vi "Profile_minus_Mean.vi"() -> (0 "New Values In":string[][](array[string])=[["Test data5"]], 1 "New Chs In":string[](array[string])=["30-10-03:New:Channel new5"])   [LabVIEW 2011]
uses:
  Results_plotter_Global.vi
  <vilib>/Analysis/NI_AALBase.lvlib
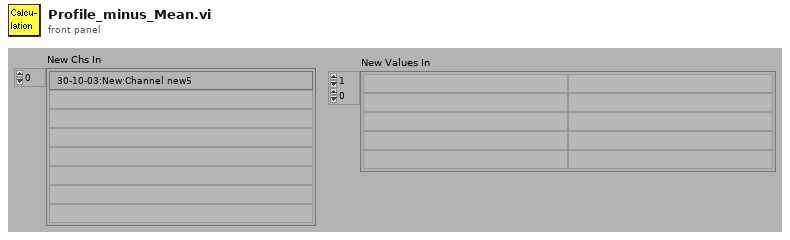
[diagram p1: front panel]
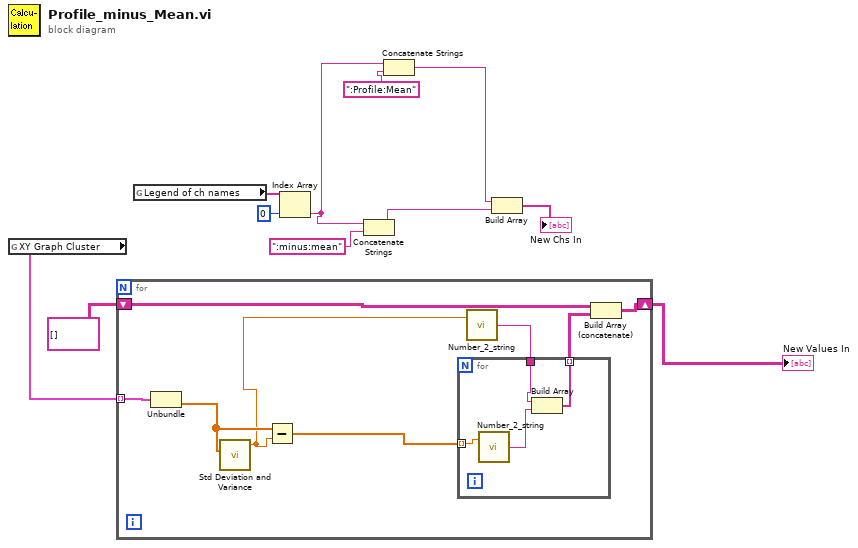
[diagram p0: block diagram]
diagram:
  n1 = global read "Results_plotter_Global.vi" "XY Graph Cluster"() -> (w9:cluster{dbl[], dbl[]}[])
  n2 = for {
    tunnel: w9 -> [w19] mode=indexing
    shift-right: [w15] -> w4
    shift-left: string[][] [] -> [w17]
    n3 = Unbundle(w19) -> (w18:dbl[])  [unwired: 1 out]
    n4 = call <vilib>:"Std Deviation and Variance.vi"("X"=w18) -> ("mean"=w14:dbl)  [unwired: 1 in, 2 out]
    n5 = Subtract(x=w18, y=w14) -> (x-y=w12:dbl[])
    n6 = call "Number_2_string.vi"("number"=w14) -> ("String"=w13:string)  [unwired: 1 in]
    n7 = for {
      tunnel: w12 -> [w23] mode=indexing
      tunnel: [w21] -> w16 mode=indexing
      tunnel: w13 -> [w20]
      n8 = call "Number_2_string.vi"("number"=w23) -> ("String"=w22:string)  [unwired: 1 in]
      n9 = Build Array(w20, w22) -> (w21:string[])
    }
    n10 = Build Array (concatenate)(w17, w16) -> (w15:string[][])
  }
  "New Values In" <- w4
  n11 = global read "Results_plotter_Global.vi" "Legend of ch names"() -> (w7:string[])
  n12 = Index Array(array=w7, index=0) -> (element=w2:string)
  n13 = Concatenate Strings(w2, ":minus:mean" ("string")) -> (w5:string)
  n14 = Concatenate Strings(w2, ":Profile:Mean" ("string")) -> (w1:string)
  n15 = Build Array(w1, w5) -> (→"New Chs In":string[])
